vi "Update MSG.vi"(8 "error in (no error)":errorcluster, 10 "Update MSG":string, 11 "MENSAJE in":refnum<class "MENSAJE.lvclass">) -> (0 "error out":errorcluster, 3 "MENSAJE out":refnum<class "MENSAJE.lvclass">)   [LabVIEW 2020, in "MENSAJE.lvlib" / "MENSAJE.lvclass"]
uses:
  MENSAJE.lvclass
  MENSAJE.lvclass/MENSAJE.ctl
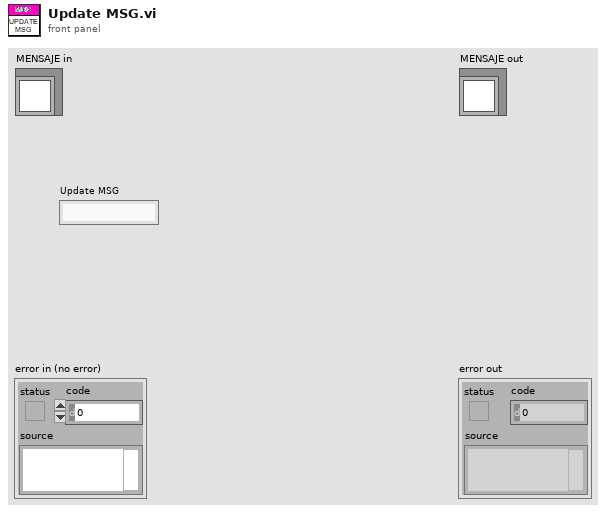
[diagram p1: front panel]
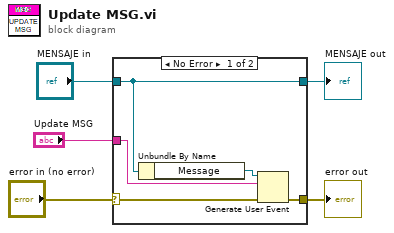
[diagram p0: block diagram]
diagram:
  n1 = case shown="No Error" "error in (no error)" {
    selector: "error in (no error)" -> [w7 w12]
    tunnel: [w6 w12] -> w4
    tunnel: [w10 w11] -> w2
    tunnel: "MENSAJE in" -> [w10 w11]
    tunnel: "Update MSG" -> [w8 _]
    frame No Error {
      n2 = Unbundle By Name(w10) -> ("Message"=w9:refnum<user-event>)
      n3 = Generate User Event(user event=w9, event data cluster=w8, error in=w7) -> (error out=w6:errorcluster)  [unwired: 1 in, 1 out]
    }
    frame Error {
    }
  }
  "error out" <- w4
  "MENSAJE out" <- w2
